vi "validate key value pair.vi"(8 "error in":errorcluster, 9 "value":string, 10 "key":string, 11 "ScaleAndLimitModule configuration in":refnum<class "ScaleAndLimitModule configuration.lvclass">) -> (0 "error out":errorcluster, 3 "ScaleAndLimitModule configuration out":refnum<class "ScaleAndLimitModule configuration.lvclass">)   [LabVIEW 2017, in "ScaleAndLimitModule configuration.lvclass"]
uses:
  ScaleAndLimitModule configuration.lvclass
  <vilib>/NI/DCAF/Tag Editor Core/control module/configuration/control module configuration.lvclass
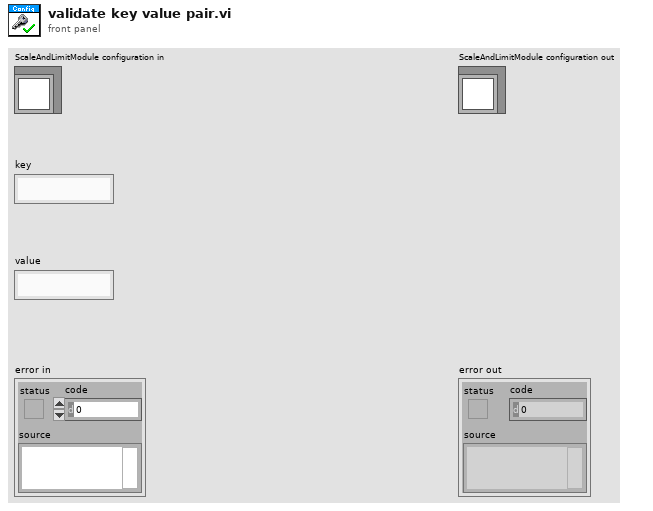
[diagram p1: front panel]
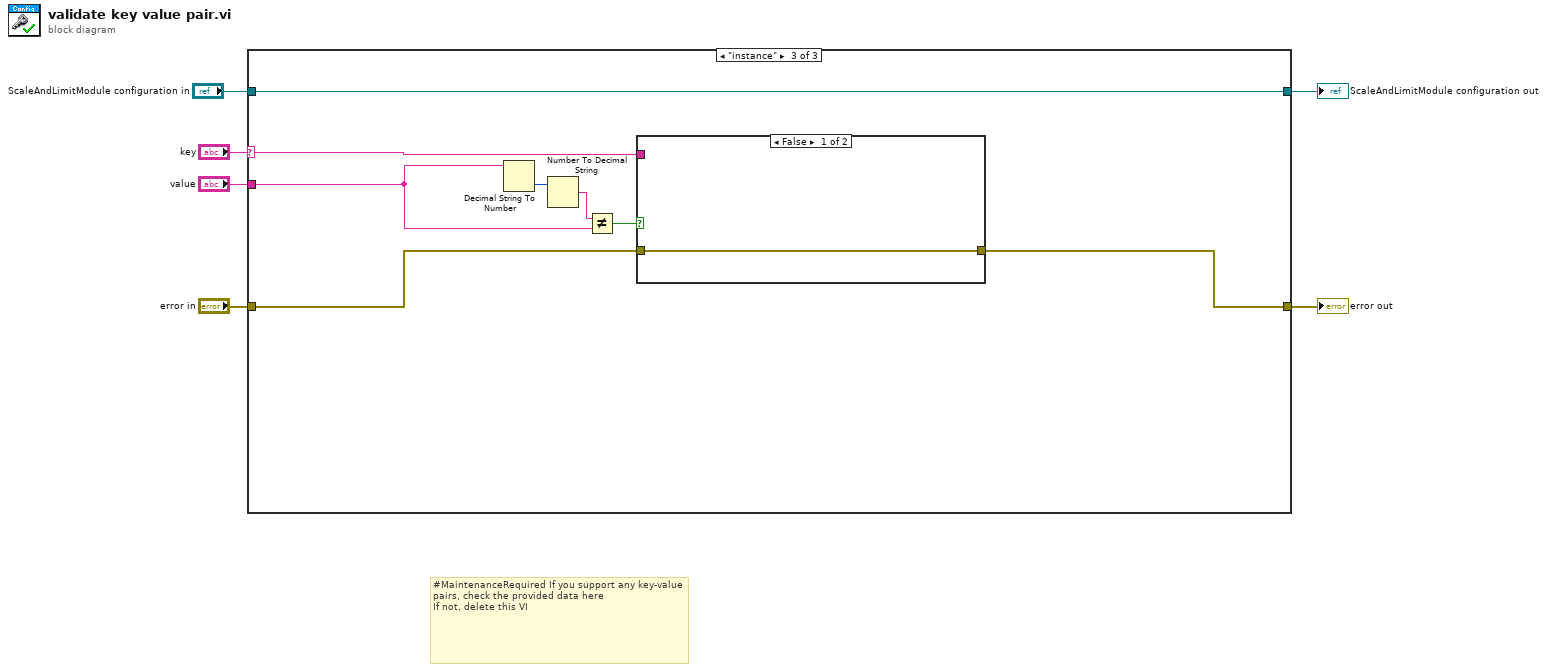
[diagram p0: block diagram]
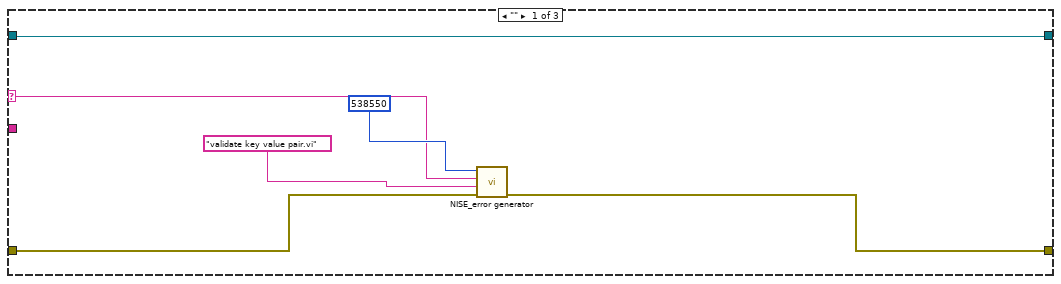
[diagram p2: hidden frame]
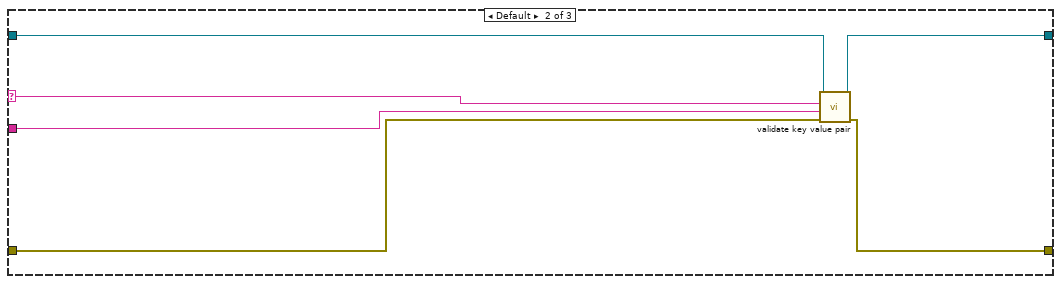
[diagram p3: hidden frame]
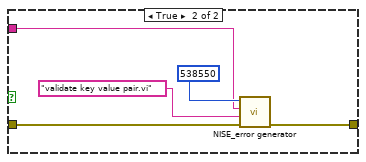
[diagram p4: hidden frame]
diagram:
  # "#MaintenanceRequired If you support any key-value pairs, check the provided data here\nIf not, delete this VI"
  n1 = case shown="\"instance\"" "key" {
    selector: "key" -> [w10 w13 w22]
    tunnel: [w8 w18 w20] -> w6
    tunnel: [w7 w17 w21] -> w5
    tunnel: "error in" -> [w9 w16 w19]
    tunnel: "value" -> [_ w15 w24]
    tunnel: "ScaleAndLimitModule configuration in" -> [w7 w14 w21]
    frame "" {
      n2 = call <vilib>:"NISE_error generator.vi"("error in"=w9, "source"="validate key value pair.vi", "append error message"=w10, "error code (0)"=538550) -> ("error out"=w8:errorcluster)  [unwired: 5 in]
    }
    frame Default {
      n3 = call-parent "validate key value pair.vi"("error in"=w16, "value"=w15, "key"=w13, "fixed channel configuration in"=w14) -> ("error out"=w18:errorcluster, "fixed channel configuration out"=w17:refnum<class "ScaleAndLimitModule configuration.lvclass">)  [unwired: 6 in]
    }
    frame "instance" {
      n4 = Decimal String To Number(string=w24) -> (number=w26:i32)  [unwired: 2 in, 1 out]
      n5 = Number To Decimal String(number=w26) -> (decimal integer string=w25:string)  [unwired: 1 in]
      n6 = Not Equal?(x=w25, y=w24) -> (x != y?=w23:bool)
      n7 = case shown="False" w23 {
        tunnel: w22 -> [_ w30]
        tunnel: [w27 w29] -> w20
        tunnel: w19 -> [w27 w28]
        frame False {
        }
        frame True {
          n8 = call <vilib>:"NISE_error generator.vi"("error in"=w28, "source"="validate key value pair.vi", "append error message"=w30, "error code (0)"=538550) -> ("error out"=w29:errorcluster)  [unwired: 5 in]
        }
      }
    }
  }
  "error out" <- w6
  "ScaleAndLimitModule configuration out" <- w5
